vi "INIT.vi"(8 "error in (no error)":errorcluster, 11 "DB_SQLite in":refnum<class "DB_SQLite.lvclass">) -> (0 "error out":errorcluster, 3 "DB_SQLite out":refnum<class "DB_SQLite.lvclass">)   [LabVIEW 2020, in "DB_SQLite.lvclass"]
uses:
  DB_SQLite/DB_SQLite.lvclass
  C:/dev/TRANCON/Classes/DB/DB.lvclass
  DB.lvclass
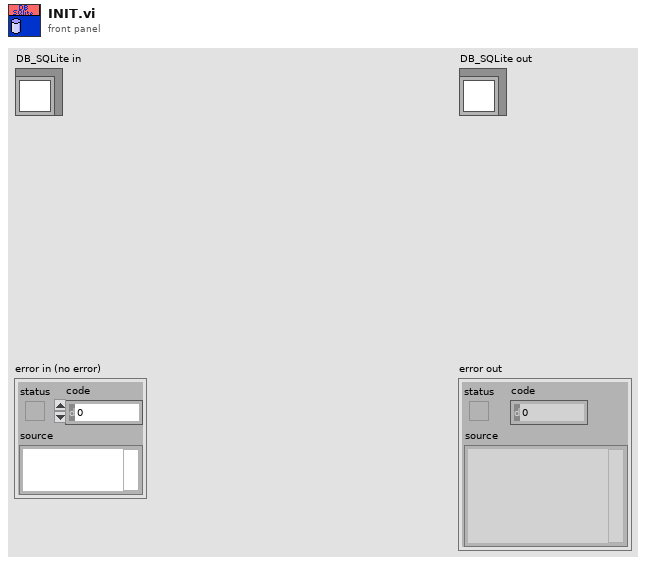
[diagram p1: front panel]
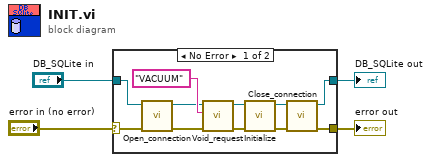
[diagram p0: block diagram]
diagram:
  n1 = case shown="No Error" "error in (no error)" {
    selector: "error in (no error)" -> [w8 w16]
    tunnel: "DB_SQLite in" -> [w6 w17]
    tunnel: [w11 w17] -> w2
    tunnel: [w10 w16] -> w1
    frame No Error {
      n2 = call-dynamic "Open_connection.vi"("error in (no error)"=w8, "DB_SQLite in"=w6) -> ("error out"=w7:errorcluster, "DB_SQLite out"=w5:refnum<class "DB_SQLite.lvclass">)  [unwired: 8 in]
      n3 = call-dynamic "Void_request.vi"("error in (no error)"=w7, "SQL request"="VACUUM" ("SQL"), "DB_SQLite in"=w5) -> ("error out"=w14:errorcluster, "DB_SQLite out"=w13:refnum<class "DB_SQLite.lvclass">)  [unwired: 7 in]
      n4 = call "Initialize.vi"("error in (no error)"=w14, "DB in"=w13) -> ("error out"=w9:errorcluster, "DB out"=w12:refnum<class "DB_SQLite.lvclass">)  [unwired: 8 in]
      n5 = call-dynamic "Close_connection.vi"("error in (no error)"=w9, "DB_SQLite in"=w12) -> ("error out"=w10:errorcluster, "DB_SQLite out"=w11:refnum<class "DB_SQLite.lvclass">)  [unwired: 8 in]
    }
    frame Error {
    }
  }
  "error out" <- w1
  "DB_SQLite out" <- w2
